vi "QueueExample1.vi"() -> ()   [LabVIEW 2024]
panel:
  out "element3":i32
  out "element2":i32
  out "element1":i32
  out "created new? 2":bool
  out "created new? 1":bool
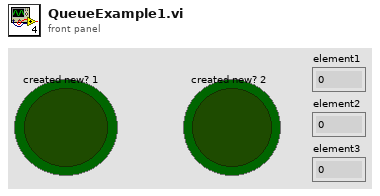
[diagram p1: front panel]
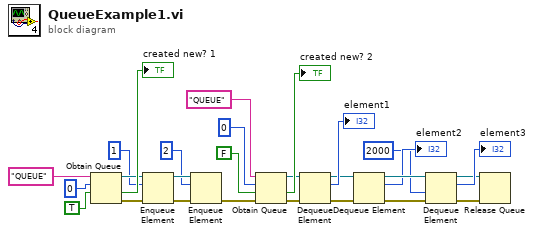
[diagram p0: block diagram]
diagram:
  n1 = Obtain Queue(name (unnamed)="QUEUE", element data type=0, create if not found? (T)=TRUE) -> (queue out=w23:refnum<queue>, created new?=→"created new? 1":bool, error out=w22:errorcluster)  [unwired: 2 in]
  n2 = Enqueue Element(queue=w23, element=1, error in (no error)=w22) -> (queue out=w20:refnum<queue>, error out=w18:errorcluster)  [unwired: 1 in, 1 out]
  n3 = Enqueue Element(queue=w20, element=2, error in (no error)=w18) -> (error out=w14:errorcluster)  [unwired: 1 in, 2 out]
  n4 = Obtain Queue(name (unnamed)="QUEUE", element data type=0, create if not found? (T)=FALSE, error in (no error)=w14) -> (queue out=w12:refnum<queue>, created new?=→"created new? 2":bool, error out=w1:errorcluster)  [unwired: 1 in]
  n5 = Dequeue Element(queue=w12, error in (no error)=w1) -> (queue out=w10:refnum<queue>, element=→"element1":i32, error out=w7:errorcluster)  [unwired: 1 in, 1 out]
  n6 = Dequeue Element(queue=w10, error in (no error)=w7) -> (queue out=w9:refnum<queue>, element=→"element2":i32, error out=w8:errorcluster)  [unwired: 1 in, 1 out]
  n7 = Dequeue Element(queue=w9, timeout in ms (-1)=2000, error in (no error)=w8) -> (queue out=w3:refnum<queue>, element=→"element3":i32, error out=w2:errorcluster)  [unwired: 1 out]
  n8 = Release Queue(queue=w3, error in (no error)=w2) -> ()  [unwired: 1 in, 3 out]
